vi "Main.vi"() -> ()   [LabVIEW 2016]
uses:
  <vilib>/event_ctls.llb/eventvkey.ctl
  <vilib>/Utility/error.llb/DialogType.ctl
  Modules/DAQ-Config/SubVIs/FGV_Cards.ctl
  SubVIs/FGV_GuideTree.ctl
  SubVIs/FGV_ThreadsManager.ctl
  Modules/DAQ-VirtualCH/SubVIs/VCH/Private/Ctrls/PSVCH_All Channels.ctl
  Modules/DAQ-Config/Controls/PSCHN_Card Para.ctl
  Modules/DAQ-Config/Controls/PSCHN_Channel Para.ctl
  Modules/DAQ-Display/PanelSplitToolkit/QueueManager.llb/CreatQueue.vi
  Modules/DAQ-Display/PanelSplitToolkit/QueueManager.llb/Remove.vi
  Modules/DAQ-Display/PanelSplitToolkit/QueueManager.llb/Insert.vi
  Modules/DAQ-Display/PanelSplitToolkit/QueueManager.llb/Destroy.vi
  Modules/DAQ-Display/PanelSplitToolkit/QueueManager.llb/Valid?.vi
panel:
  in  "Tree":string[](tree)
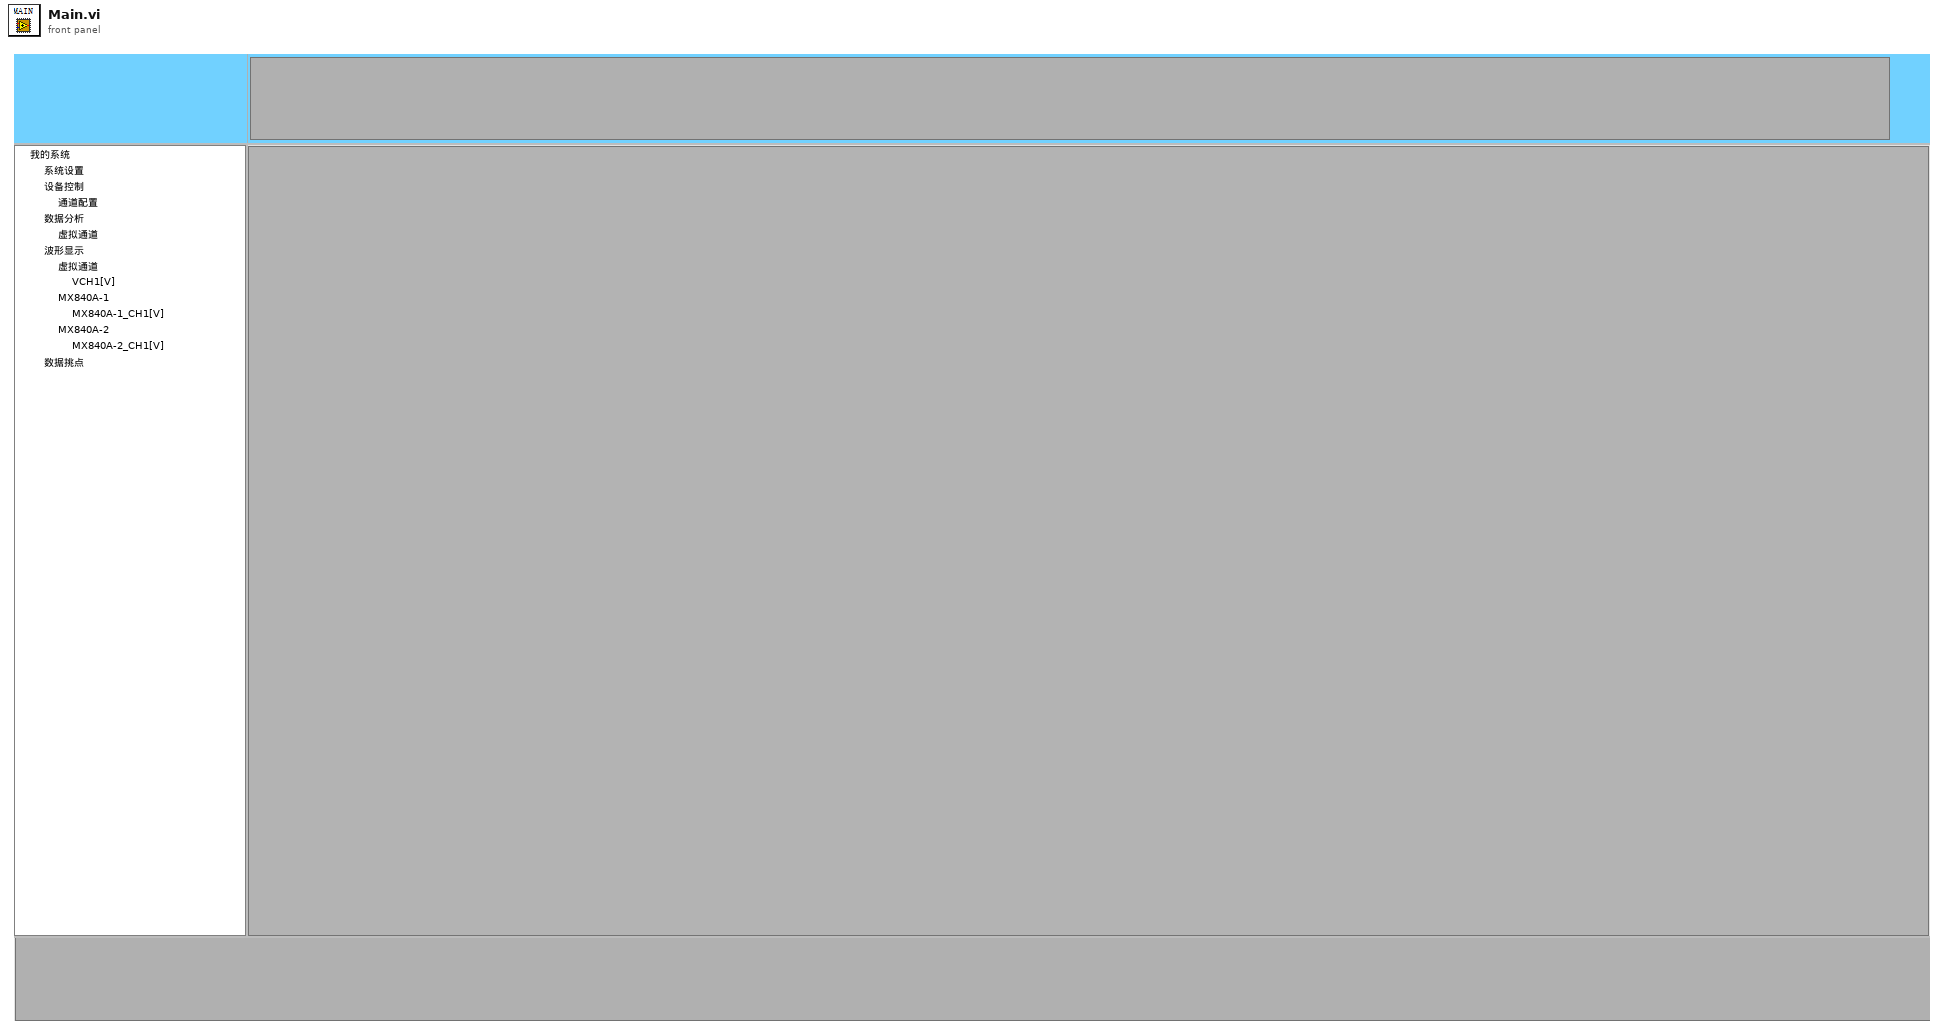
[diagram p1: front panel]
types:
  T1 = cluster{"error":errorcluster, "LocalQ":cluster{"LQName":string, "LQEvent":string, "LQData":variant}, "HighQ":cluster{"HQName":string, "HQEvent":string, "HQData":variant}, "SubPnl_Main":refnum<vi>, "Tree":refnum<vi>}
  T2 = cluster{"Main Queue":string, "DAQ Queue":string, "ANA Queue":string, "CUI Queue":string, "Q-FocusList":string, "Q-Toolbar":string, "Q-Config":string}
  T3 = typedef "eventvkey.ctl" = enum16{"ASCII", "Enter", "Return", "Shift", "Ctrl", "Alt", "Cmd", "Opt", "Caps", "NumLock", "Clear", "Break", "Up", "Down", "Left", "Right", "Insert", "Delete", "Home", "End", "PageUp", "PageDown", "Escape", "Help", "Pause", "ScrollLock", "F1", "F2", "F3", "F4", "F5", "F6", "F7", "F8", "F9", "F10", "F11", "F12", "F13", "F14", "F15", "F16", "F17", "F18", "F19", "F20", "F21", "F22", "F23", "F24", "Play", "VolumeUp", "VolumeDown", "Mute", "Two Byte Char"}
  T4 = cluster{"data name":string, "drag data":variant}[]
  T5 = typedef "FGV_Cards.ctl" = enum16{"Initlize", "Set_DAQCards", "Set_VCHCards", "Get_DAQCards", "Get_VCHCards", "Get_ALLUsing"}
  T6 = typedef "FGV_GuideTree.ctl" = enum16{"SetTree*", "GetTree*", "InitlizeTree", "AddCards"}
  T7 = typedef "FGV_ThreadsManager.ctl" = enum16{"Load Threads", "GetVI*", "Other"}
  T8 = typedef "PSVCH_All Channels.ctl" = cluster{"Card Name":string, "Channels Tag":string[], "Channels Name":string[], "Unit":string[]}
  T9 = typedef "PSCHN_Card Para.ctl" = cluster{"Module Type":string, "Module Name":string, "ModuSN":string, "ModuIP":string, "Used?":bool, "Connected":bool, "Timing*":cluster{"Sample Rate":dbl}, "Channels":T10[]}
  T10 = typedef "PSCHN_Channel Para.ctl" = cluster{"CHTag*":string, "Used?*":bool, "CHName":string, "Unit":string, "斜率":dbl, "截距":dbl}
  T11 = typedef "DialogType.ctl" = u16
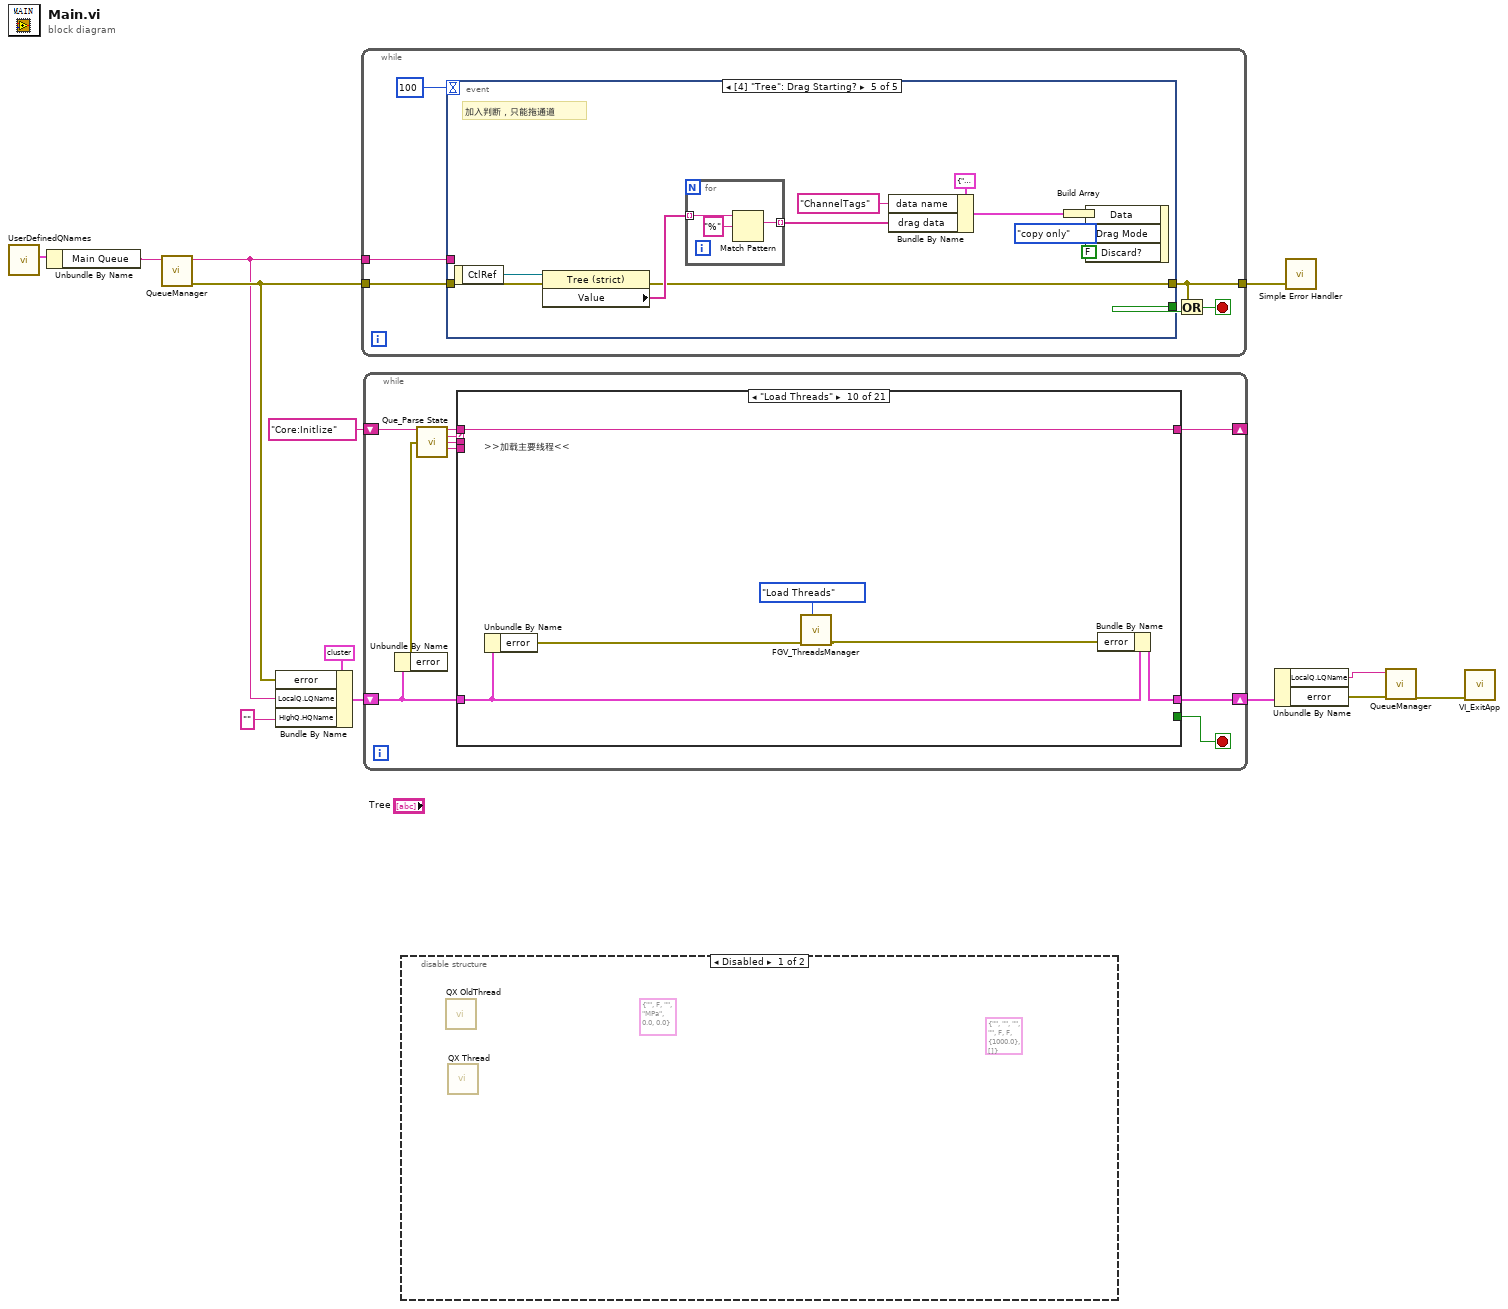
[diagram p0: block diagram]
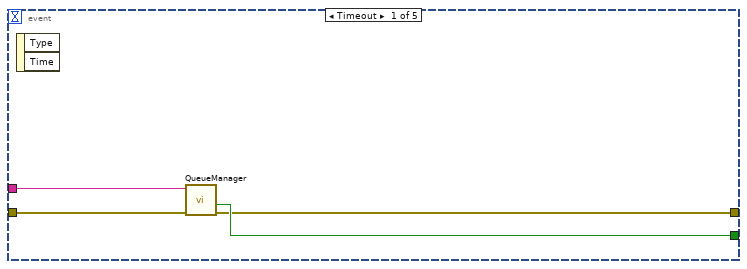
[diagram p3: hidden frame]
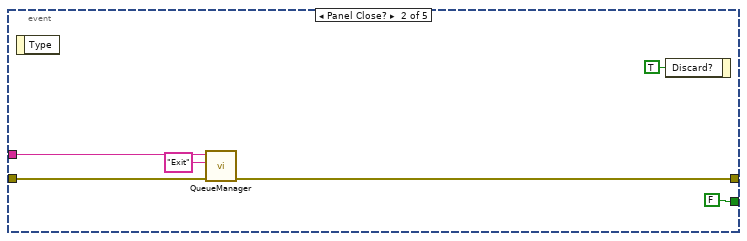
[diagram p4: hidden frame]
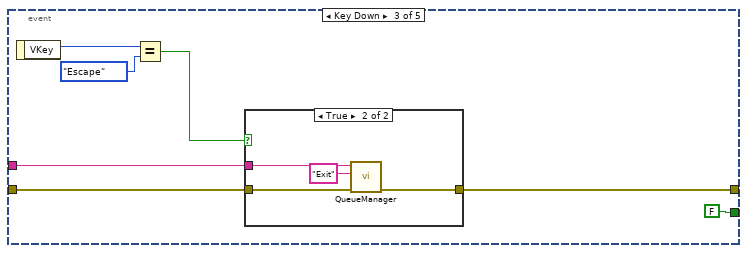
[diagram p5: hidden frame]
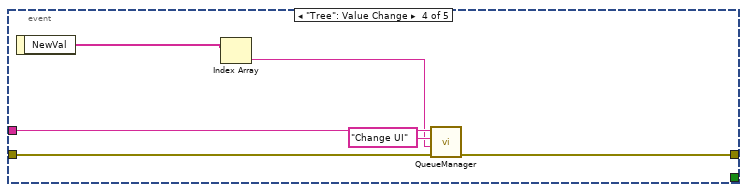
[diagram p7: hidden frame]
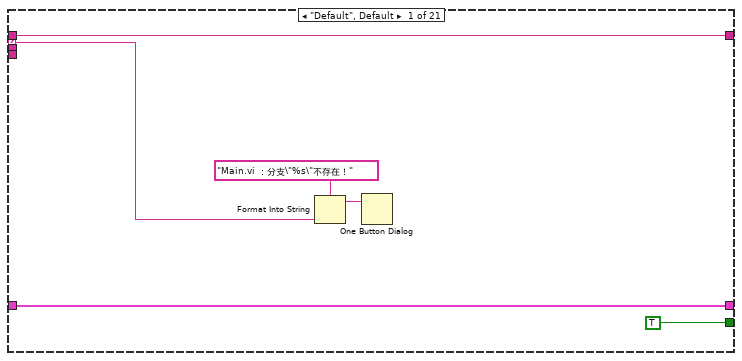
[diagram p8: hidden frame]
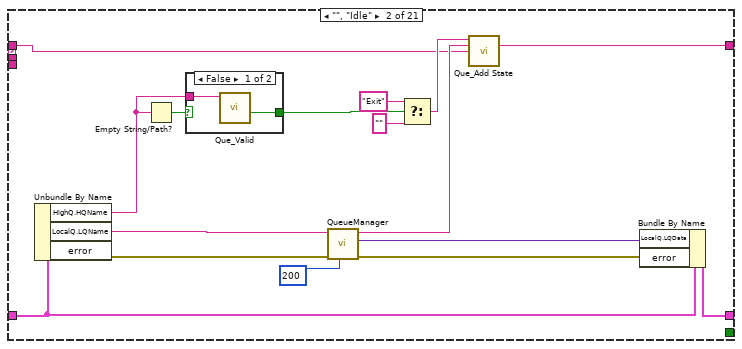
[diagram p9: hidden frame]
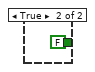
[diagram p10: hidden frame]
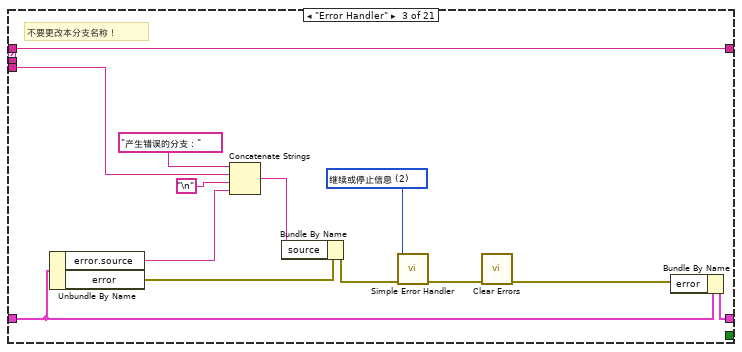
[diagram p11: hidden frame]
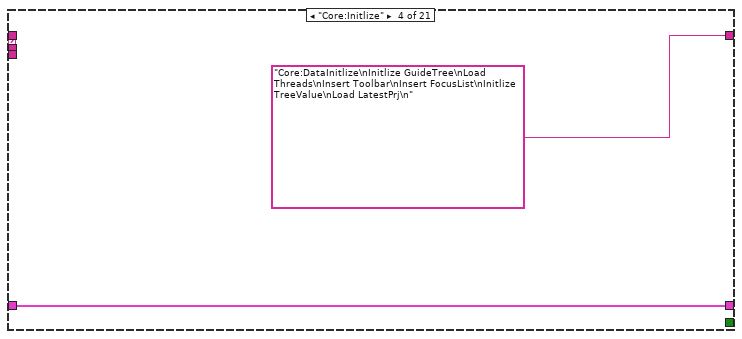
[diagram p12: hidden frame]
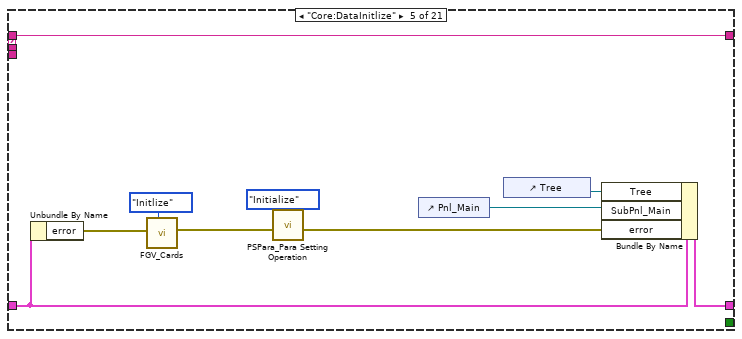
[diagram p13: hidden frame]
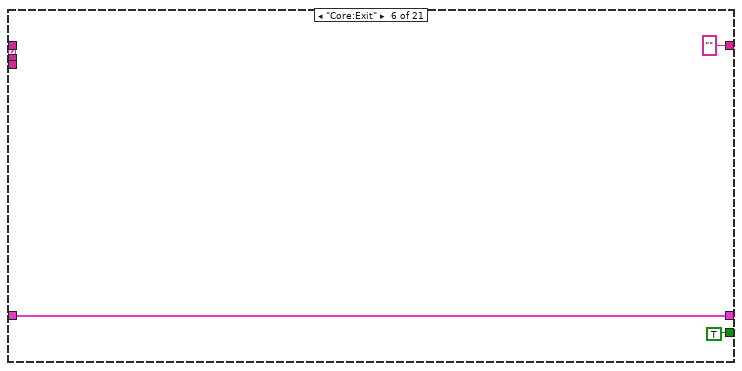
[diagram p14: hidden frame]
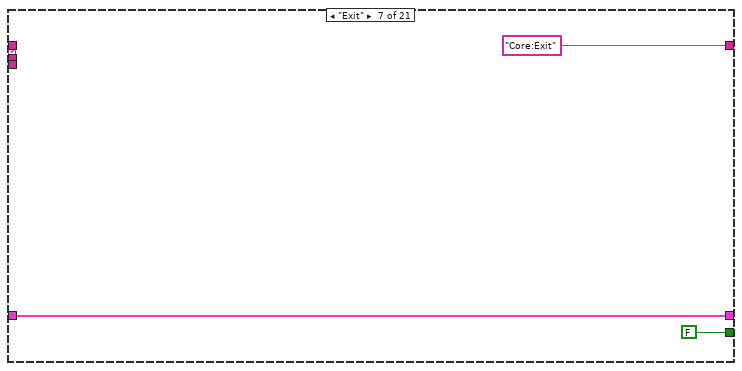
[diagram p15: hidden frame]
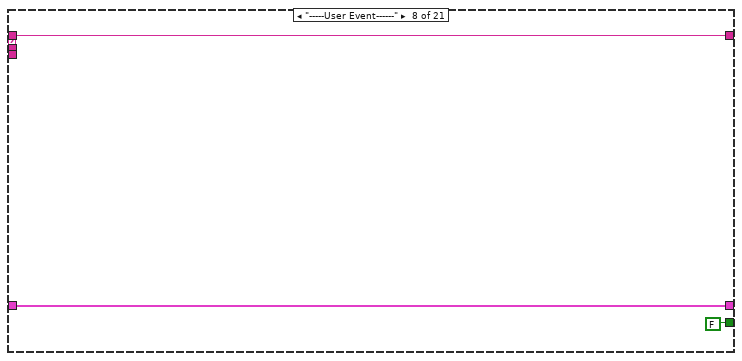
[diagram p16: hidden frame]
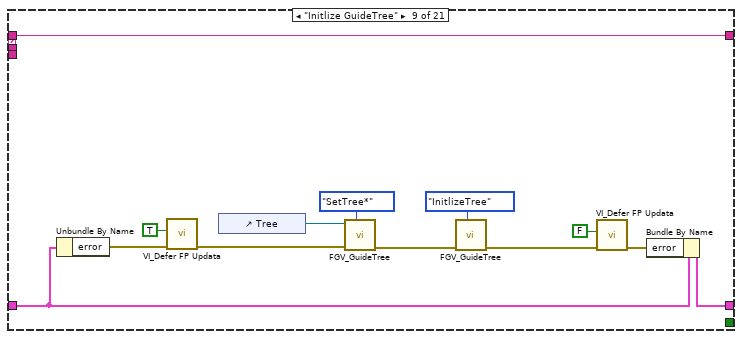
[diagram p17: hidden frame]
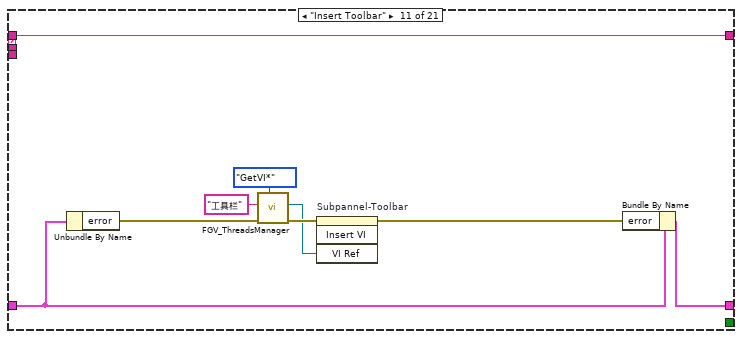
[diagram p18: hidden frame]
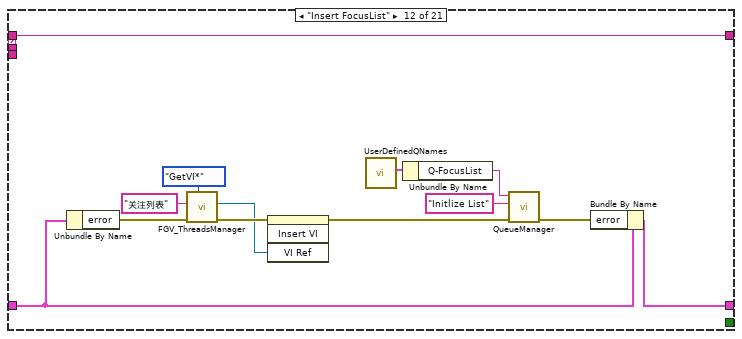
[diagram p19: hidden frame]
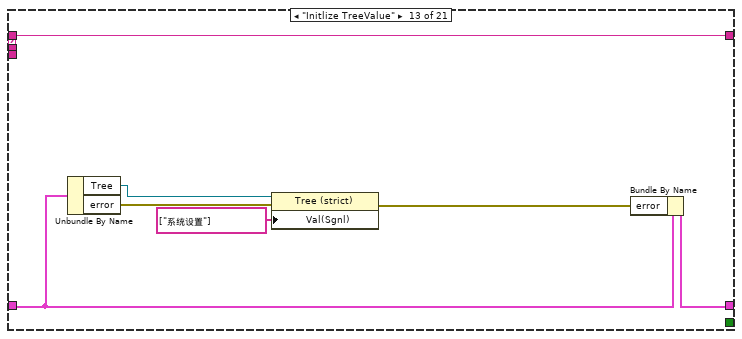
[diagram p20: hidden frame]
diagram:
  n1 = call "UserDefinedQNames.vi"() -> ("All Queues"=w3:T2)  [unwired: 11 in]
  n2 = Unbundle By Name(w3) -> ("Main Queue"=w2:string)
  n3 = call-poly "QueueManager.vi"("QueueName"=w2) -> ("error out"=w7:errorcluster, "QueueName out"=w5:string)  [unwired: 9 in]
  n4 = Bundle By Name(cluster=T1 {"error"={"status"=FALSE, "code"=0, "source"=""}, "LocalQ"={"LQName"="", "LQEvent"="", "LQData"=variant}, "HighQ"={"HQName"="", "HQEvent"="", "HQData"=variant}, "SubPnl_Main"=refnum, "Tree"=refnum} ("TmpData"), "error"=w7, "LocalQ.LQName"=w5, "HighQ.HQName"="" ("Caller")) -> (w9:T1)
  n5 = while {
    tunnel: w7 -> [w18]
    tunnel: w5 -> [w19]
    tunnel: [w15] -> w10
    stop <- w16 stop-if-true
    n6 = event shown="[4] \"Tree\": Drag Starting?" {
      selector: _ -> [_ _ _ _ _]
      dyn-events: _ -> [_ _ _ _ _]
      timeout: 100 -> [_ _ _ _ _]
      tunnel: [w21 FALSE FALSE _ _] -> w17
      tunnel: w19 -> [w23 w28 w35 w45 _]
      tunnel: w18 -> [w22 w27 w34 w47 w50]
      tunnel: [w20 w26 w33 w46 w49] -> w15
      event Timeout {
        n7 = event-data() -> ()  [unwired: 1 in, 2 out]
        n8 = call-poly "QueueManager.vi"("error in (no error)"=w22, "Queue Name(unamed)"=w23) -> ("error out"=w20:errorcluster, "Not Exist?"=w21:bool)  [unwired: 8 in]
      }
      event Panel Close? {
        n9 = event-data() -> ()  [unwired: 1 in, 1 out]
        n10 = call-poly "QueueManager.vi"("error in"=w27, "Event"="Exit", "QueueName"=w28) -> ("error out"=w26:errorcluster)  [unwired: 7 in, 1 out]
        n11 = event-data("Discard?"=TRUE ("放弃？")) -> ()  [unwired: 1 in, 1 out]
      }
      event Key Down {
        n12 = event-data() -> ("VKey"=w32:T3)  [unwired: 1 in]
        n13 = Equal?(x=w32, y=eventvkey."Escape" ("V键")) -> (x = y?=w30:bool)
        n14 = case shown="True" w30 {
          tunnel: w35 -> [_ w41]
          tunnel: w34 -> [w37 w40]
          tunnel: [w37 w39] -> w33
          frame False {
          }
          frame True {
            n15 = call-poly "QueueManager.vi"("error in"=w40, "Event"="Exit", "QueueName"=w41) -> ("error out"=w39:errorcluster)  [unwired: 7 in, 1 out]
          }
        }
      }
      event "Tree": Value Change {
        n16 = event-data() -> ("NewVal"=w43:string[])  [unwired: 1 in]
        n17 = Index Array(array=w43) -> (element=w42:string)  [unwired: 1 in]
        n18 = call-poly "QueueManager.vi"("error in"=w47, "Data"=w42, "Event"="Change UI", "QueueName"=w45) -> ("error out"=w46:errorcluster)  [unwired: 6 in, 1 out]
      }
      event "Tree": Drag Starting? {
        # "加入判断，只能拖通道"
        n19 = event-data() -> ("CtlRef"=w52:refnum<vi>)  [unwired: 1 in]
        n20 = property class="Tree (strict)"(reference=w52, error in=w50) -> (error out=w49:errorcluster, "Value"=w51:string[])  [unwired: 1 out]
        n21 = for {
          tunnel: [w61] -> w48 mode=indexing
          tunnel: w51 -> [w59] mode=indexing
          n22 = Match Pattern(string=w59, regular expression="%" ("正则表达式")) -> (after substring=w61:string)  [unwired: 1 in, 3 out]
        }
        n23 = Bundle By Name(cluster=cluster{"data name":string, "drag data":variant} {"data name"="", "drag data"=variant}, "data name"="ChannelTags", "drag data"=w48) -> (w55:cluster{"data name":string, "drag data":variant})
        n24 = Build Array(w55) -> (w54:T4)
        n25 = event-data("Data"=w54, "Drag Mode"=enum32{"copy or move", "copy only", "move only"}."copy only" ("拖曳模式"), "Discard?"=FALSE ("放弃？")) -> ()  [unwired: 1 in, 1 out]
      }
    }
    n26 = Or(x=w15, y=w17) -> (x .or. y?=w16:bool)
  }
  n27 = while {
    shift-right: [w65] -> w11
    shift-left: w9 -> [w66]
    shift-right: [w64] -> _
    shift-left: "Core:Initlize" -> [w71]
    stop <- w68 stop-if-true
    n28 = Unbundle By Name(w66) -> ("error"=w67:errorcluster)
    n29 = call "Que_Parse State.vi"("State Queue"=w71, "Error In (no error)"=w67) -> ("Remaining States"=w70:string, "Current State"=w69:string, "Arguments"=w63:string, "PreState"=w62:string)  [unwired: 10 in]
    n30 = case shown="\"Load Threads\"" w69 {
      selector: w69 -> [w75 _ _ _ _ _ _ _ _ _ _ _ _ _ _ _ _ _ _ _ _]
      tunnel: w70 -> [w76 w78 w109 _ w121 _ _ w128 w143 w149 w158 w171 w178 w183 w202 w203 w213 w214 w218 w234 w251]
      tunnel: w63 -> [_ _ _ _ _ _ _ _ _ _ _ _ _ _ _ _ _ _ _ _ _]
      tunnel: [TRUE _ _ _ _ TRUE FALSE FALSE _ _ _ _ _ _ _ _ _ _ _ _ _] -> w68
      tunnel: w66 -> [w77 w88 w106 w111 w118 w123 w126 w129 w141 w148 w157 w170 w177 w181 w201 w204 w212 w215 w220 w236 w253]
      tunnel: [w77 w92 w105 w111 w117 w123 w126 w129 w140 w147 w155 w169 w176 w179 w200 w204 w212 w215 w219 w235 w252] -> w65
      tunnel: [w76 w90 w109 "Core:DataInitlize\nInitlize GuideTree\nLoad Threads\nInsert Toolbar\nInsert FocusList\nInitlize TreeValue\nLoad LatestPrj\n" w121 "" ("Remaining States") "Core:Exit" ("Remaining States") w128 w143 w149 w158 w171 w178 w183 w202 w203 w213 w214 w217 w233 w250] -> w64
      tunnel: w62 -> [_ _ w103 _ _ _ _ _ _ _ _ _ _ _ _ _ _ _ _ _ _]
      frame "Default", Default {
        n31 = Format Into String(format string="Main.vi ：分支\"%s\"不存在！" ("格式字符串"), w75) -> (resulting string=w74:string)  [unwired: 2 in, 1 out]
        n32 = One Button Dialog(message=w74) -> ()  [unwired: 1 in, 1 out]
      }
      frame "", "Idle" {
        n33 = Unbundle By Name(w88) -> ("HighQ.HQName"=w82:string, "LocalQ.LQName"=w87:string, "error"=w86:errorcluster)
        n34 = Empty String/Path?(string/path=w82) -> (empty?=w85:bool)
        n35 = case shown="False" w85 {
          tunnel: [w95 FALSE ("Not Exist?")] -> w84
          tunnel: w82 -> [w94 _]
          frame False {
            n36 = call "Que_Valid.vi"("Queue Name(unamed)"=w94) -> ("Not Exist?"=w95:bool)  [unwired: 9 in, 1 out]
          }
          frame True {
          }
        }
        n37 = call-poly "QueueManager.vi"("Time out(-1)"=200, "error in (no error)"=w86, "Queue Name"=w87) -> ("error out"=w93:errorcluster, "Data"=w91:variant, "Event"=w79:string)  [unwired: 5 in, 1 out]
        n38 = Select(t="Exit" ("Event"), s=w84, f="") -> (s? t:f=w80:string)
        n39 = call "Que_Add State.vi"("State(s) in Front (\"\")"=w80, "State(s) in (\"\")"=w79, "State(s) at Back (\"\")"=w78) -> ("States Out"=w90:string)  [unwired: 12 in]
        n40 = Bundle By Name(cluster=w88, "LocalQ.LQData"=w91, "error"=w93) -> (w92:T1)
      }
      frame "Error Handler" {
        w104 = T11 2 items=["无对话框", "确定信息", "继续或停止信息", "确定信息＋警告", "继续/停止+警告"] ("type of dialog (OK msg:1)")
        # "不要更改本分支名称！"
        n41 = Unbundle By Name(w106) -> ("error.source"=w97:string, "error"=w99:errorcluster)
        n42 = Concatenate Strings("产生错误的分支：" ("字符串"), w103, "\n", w97) -> (w100:string)
        n43 = Bundle By Name(cluster=w99, "source"=w100) -> (w98:errorcluster)
        n44 = call <vilib>:"Simple Error Handler.vi"("type of dialog (OK msg:1)"=w104, "error in (no error)"=w98) -> ("error out"=w107:errorcluster)  [unwired: 3 in, 4 out]
        n45 = call <vilib>:"Clear Errors.vi"("error in (no error)"=w107) -> ("error out"=w108:errorcluster)  [unwired: 5 in, 1 out]
        n46 = Bundle By Name(cluster=w106, "error"=w108) -> (w105:T1)
      }
      frame "Core:Initlize" {
      }
      frame "Core:DataInitlize" {
        n47 = Unbundle By Name(w118) -> ("error"=w119:errorcluster)
        n48 = call "FGV_Cards.vi"("Action"=FGV_Cards."Initlize", "error in (no error)"=w119) -> ("error out"=w114:errorcluster)  [unwired: 8 in, 1 out]
        n49 = call "PSPara_Para Setting Operation.vi"("Operation"=enum16{"Set Value", "Get Value", "Initialize"}."Initialize", "error in (no error)"=w114) -> ("error out"=w113:errorcluster)  [unwired: 8 in, 1 out]
        n50 = control-ref of="Pnl_Main"() -> (w112:refnum<vi>)
        n51 = control-ref of="Tree"() -> (w116:refnum<vi>)
        n52 = Bundle By Name(cluster=w118, "Tree"=w116, "SubPnl_Main"=w112, "error"=w113) -> (w117:T1)
      }
      frame "Core:Exit" {
      }
      frame "Exit" {
      }
      frame "-----User Event------" {
      }
      frame "Initlize GuideTree" {
        n53 = Unbundle By Name(w141) -> ("error"=w135:errorcluster)
        n54 = call "VI_Defer FP Updata.vi"("error in"=w135, "Defer updata?"=TRUE) -> ("错误输出"=w134:errorcluster)  [unwired: 8 in, 1 out]
        n55 = control-ref of="Tree"() -> (w137:refnum<vi>)
        n56 = call "FGV_GuideTree.vi"("Action"=FGV_GuideTree."SetTree*", "error in"=w134, "Tree*"=w137) -> ("error out"=w139:errorcluster)  [unwired: 7 in, 1 out]
        n57 = call "FGV_GuideTree.vi"("Action"=FGV_GuideTree."InitlizeTree", "error in"=w139) -> ("error out"=w132:errorcluster)  [unwired: 8 in, 1 out]
        n58 = call "VI_Defer FP Updata.vi"("error in"=w132, "Defer updata?"=FALSE) -> ("错误输出"=w131:errorcluster)  [unwired: 8 in, 1 out]
        n59 = Bundle By Name(cluster=w141, "error"=w131) -> (w140:T1)
      }
      frame "Load Threads" {
        # ">>加载主要线程<<"
        n60 = Unbundle By Name(w148) -> ("error"=w146:errorcluster)
        n61 = call "FGV_ThreadsManager.vi"("Action"=FGV_ThreadsManager."Load Threads", "error in"=w146) -> ("error out"=w144:errorcluster)  [unwired: 8 in, 1 out]
        n62 = Bundle By Name(cluster=w148, "error"=w144) -> (w147:T1)
      }
      frame "Insert Toolbar" {
        n63 = Unbundle By Name(w157) -> ("error"=w151:errorcluster)
        n64 = call "FGV_ThreadsManager.vi"("Action"=FGV_ThreadsManager."GetVI*", "error in"=w151, "Tag"="工具栏") -> ("error out"=w152:errorcluster, "Vi*"=w150:refnum<vi>)  [unwired: 7 in]
        n65 = invoke on="Subpannel-Toolbar" class="SubPnl" method="Insert VI"(error in=w152, "VI Ref"=w150) -> (error out=w156:errorcluster)  [unwired: 2 in, 3 out]
        n66 = Bundle By Name(cluster=w157, "error"=w156) -> (w155:T1)
      }
      frame "Insert FocusList" {
        n67 = Unbundle By Name(w170) -> ("error"=w166:errorcluster)
        n68 = call "FGV_ThreadsManager.vi"("Action"=FGV_ThreadsManager."GetVI*", "error in"=w166, "Tag"="关注列表") -> ("error out"=w167:errorcluster, "Vi*"=w165:refnum<vi>)  [unwired: 7 in]
        n69 = invoke on="Pannel_FocusListUI" class="SubPnl" method="Insert VI"(error in=w167, "VI Ref"=w165) -> (error out=w163:errorcluster)  [unwired: 2 in, 3 out]
        n70 = call "UserDefinedQNames.vi"() -> ("All Queues"=w161:T2)  [unwired: 11 in]
        n71 = Unbundle By Name(w161) -> ("Q-FocusList"=w160:string)
        n72 = call-poly "QueueManager.vi"("error in"=w163, "Event"="Initlize List", "QueueName"=w160) -> ("error out"=w162:errorcluster)  [unwired: 7 in, 1 out]
        n73 = Bundle By Name(cluster=w170, "error"=w162) -> (w169:T1)
      }
      frame "Initlize TreeValue" {
        n74 = Unbundle By Name(w177) -> ("Tree"=w175:refnum<vi>, "error"=w174:errorcluster)
        n75 = property class="Tree (strict)"(reference=w175, error in=w174, "Val(Sgnl)"=string[] ["系统设置"] ("值(信号)")) -> (error out=w173:errorcluster)  [unwired: 1 out]
        n76 = Bundle By Name(cluster=w177, "error"=w173) -> (w176:T1)
      }
      frame "Load LatestPrj" {
        # "加载上一次打开的项目配置"
        n77 = Unbundle By Name(w181) -> ("error"=w182:errorcluster)
        n78 = disable-structure shown="启用" {
          disable-tunnel: w182 -> [w188 _]
          disable-tunnel: [w184 _] -> w180
          frame Enabled {
            n79 = call "PrjPath_Read.vi"("error in (no error)"=w188) -> ("error out"=w187:errorcluster, "Valid"=w186:bool, "Path"=w185:path)  [unwired: 7 in]
            n80 = case shown="True" w186 {
              tunnel: w187 -> [w189 w192]
              tunnel: w185 -> [_ w191]
              tunnel: [w189 w190] -> w184
              frame False {
              }
              frame True {
                n81 = call "Project Open.vi"("error in"=w192, "File Path"=w191) -> ("error out"=w190:errorcluster)  [unwired: 9 in]
              }
            }
          }
          frame Disabled {
          }
        }
        n82 = Bundle By Name(cluster=w181, "error"=w180) -> (w179:T1)
      }
      frame "Change UI" {
        w197 = ""  # Tag
        # ">>根据导航树Tag切换界面<<"
        n83 = Unbundle By Name(w201) -> ("SubPnl_Main"=w193:refnum<vi>, "LocalQ.LQData"=w199:variant, "error"=w198:errorcluster)
        n84 = Variant To Data(error in=w198, type=w197, Variant=w199) -> (data=w195:string, error out=w196:errorcluster)
        n85 = call "ChangeUI.vi"("error in (no error)"=w196, "TreeTag"=w195, "SubPnl*"=w193) -> ("error out"=w194:errorcluster)  [unwired: 8 in]
        n86 = Bundle By Name(cluster=w201, "error"=w194) -> (w200:T1)
      }
      frame "----------Tree------------" {
      }
      frame "Tree : Updata CHs" {
        # "配置变更时刷新导航树上的通道"
        n87 = Unbundle By Name(w212) -> ("error"=w209:errorcluster)
        n88 = call "VI_Defer FP Updata.vi"("error in"=w209, "Defer updata?"=TRUE) -> ("错误输出"=w208:errorcluster)  [unwired: 8 in, 1 out]
        n89 = call "FGV_GuideTree.vi"("Action"=FGV_GuideTree."AddCards", "error in"=w208) -> ("error out"=w206:errorcluster)  [unwired: 8 in, 1 out]
        n90 = call "VI_Defer FP Updata.vi"("error in"=w206, "Defer updata?"=FALSE) -> ("错误输出"=w205:errorcluster)  [unwired: 8 in, 1 out]
        n91 = Bundle By Name(cluster=w212, "error"=w205) -> ()  [unwired: 1 out]
      }
      frame "---------线程通讯----------" {
      }
      frame "COM : VCH_CFG Updata" {
        # "VCH线程发来的Cards信息"
        n92 = Unbundle By Name(w220) -> ("LocalQ.LQData"=w229:variant, "error"=w228:errorcluster)
        n93 = Variant To Data(error in=w228, type=T8 {"Card Name"="", "Channels Tag"=[], "Channels Name"=[], "Unit"=[]} ("VCHList"), Variant=w229) -> (data=w225:T8, error out=w226:errorcluster)
        n94 = call "Convert VCH to Card.vi"("VCHList"=w225) -> ("Card"=w224:T9)  [unwired: 10 in]
        n95 = Build Array(w224) -> (w223:T9[])
        n96 = call "FGV_Cards.vi"("Action"=FGV_Cards."Set_VCHCards", "error in (no error)"=w226, "Cards in"=w223) -> ("error out"=w221:errorcluster)  [unwired: 7 in, 1 out]
        n97 = call "Que_Add State.vi"("State(s) in (\"\")"=w218, "State(s) at Back (\"\")"="Tree : Updata CHs\nCOM : UpdataGraphCH" ("State(s) at Back (\"\")")) -> ("States Out"=w217:string)  [unwired: 13 in]
        n98 = Bundle By Name(cluster=w220, "error"=w221) -> (w219:T1)
      }
      frame "COM : DAQ_CFG Updata" {
        # "DAQ配置线程发来的Cards信息"
        n99 = Unbundle By Name(w236) -> ("LocalQ.LQData"=w241:variant, "error"=w240:errorcluster)
        n100 = Variant To Data(error in=w240, type=T9[] [{"Module Type"="", "Module Name"="QX111", "ModuSN"="", "ModuIP"="", "Used?"=TRUE, "Connected"=FALSE, "Timing*"={"Sample Rate"=1000.0}, "Channels"=[{"CHTag*"="CH1", "Used?*"=TRUE, "CHName"="11", "Unit"="MPa", "斜率"=0.0, "截距"=0.0}, {"CHTag*"="CH2", "Used?*"=TRUE, "CHName"="2", "Unit"="MPa", "斜率"=0.0, "截距"=0.0}]}] ("Cards in"), Variant=w241) -> (data=w230:T9[], error out=w239:errorcluster)
        n101 = call "FGV_Cards.vi"("Action"=FGV_Cards."Set_DAQCards", "error in (no error)"=w239, "Cards in"=w230) -> ("error out"=w237:errorcluster)  [unwired: 7 in, 1 out]
        n102 = call "Que_Add State.vi"("State(s) in (\"\")"=w234, "State(s) at Back (\"\")"="Tree : Updata CHs\nCOM : UpdataGraphCH" ("State(s) at Back (\"\")")) -> ("States Out"=w233:string)  [unwired: 13 in]
        n103 = Bundle By Name(cluster=w236, "error"=w237) -> (w235:T1)
      }
      frame "COM : UpdataGraphCH" {
        # "配置变更后，向所有波形图vi发指令，更新通道信息"
        n104 = Unbundle By Name(w253) -> ("error"=w245:errorcluster)  [unwired: 1 out]
        n105 = call "UserDefinedQNames.vi"() -> ("All Queues"=w248:T2)  [unwired: 11 in]
        n106 = Unbundle By Name(w248) -> ("CUI Queue"=w247:string)
        n107 = Bundle By Name(cluster=cluster{"Event":string, "Data":variant} {"Event"="", "Data"=variant} ("Send"), "Event"="Rec : UpdataConfig") -> (w242:cluster{"Event":string, "Data":variant})
        n108 = call-poly "QueueManager.vi"("error in"=w245, "Data"=w242, "Event"="SendToAllPanels", "QueueName"=w247) -> ("error out"=w246:errorcluster)  [unwired: 6 in, 1 out]
        n109 = call "Que_Add State.vi"("State(s) in (\"\")"=w251) -> ("States Out"=w250:string)  [unwired: 14 in]
        n110 = Bundle By Name(cluster=w253, "error"=w246) -> (w252:T1)
      }
    }
  }
  n111 = disable-structure shown="Disabled" {
    frame Disabled {
      (unwired) T9 {"Module Type"="", "Module Name"="", "ModuSN"="", "ModuIP"="", "Used?"=FALSE, "Connected"=FALSE, "Timing*"={"Sample Rate"=1000.0}, "Channels"=[]} ("Card")
      (unwired) T10 {"CHTag*"="", "Used?*"=FALSE, "CHName"="", "Unit"="MPa", "斜率"=0.0, "截距"=0.0} ("Channel")
      n112 = call "QX OldThread.vi"() -> ()  [unwired: 12 in]
      n113 = call "QX Thread.vi"() -> ()  [unwired: 12 in]
    }
    frame Enabled {
    }
  }
  n114 = Unbundle By Name(w11) -> ("LocalQ.LQName"=w8:string, "error"=w12:errorcluster)
  n115 = call <vilib>:"Simple Error Handler.vi"("error in (no error)"=w10) -> ()  [unwired: 4 in, 5 out]
  n116 = call-poly "QueueManager.vi"("error in (no error)"=w12, "QueeuName"=w8) -> ("error out"=w1:errorcluster)  [unwired: 9 in]
  n117 = call "VI_ExitApp.vi"("错误输入（无错误）"=w1) -> ()  [unwired: 10 in, 1 out]
